vi "Project Directory Change Callback.vi"(4 "Variant":variant, 5 "Event Data":cluster{"sender":refnum<k24>, "e":refnum<k24>}, 6 "Control Ref":refnum<k24>, 7 "Event Common Data":T1) -> ()   [LabVIEW 2015, in "Editor.lvclass"]
uses:
  Editor.lvclass
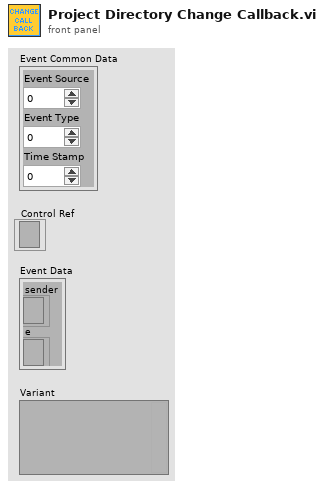
[diagram p1: front panel]
types:
  T1 = cluster{"Event Source":i32, "Event Type":u32, "Time Stamp":u32}
  T2 = cluster{"Event":enum16{"Changed", "Created", "Deleted", "Renamed", "Error"}, "Explorer Tree":refnum<vi>, "Path":path}
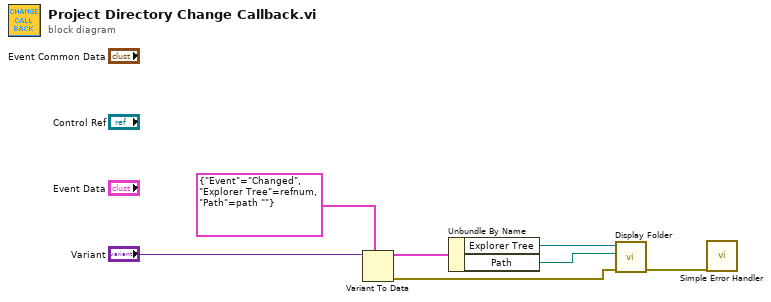
[diagram p0: block diagram]
diagram:
  n1 = Variant To Data(type=T2 {"Event"=enum."Changed", "Explorer Tree"=refnum, "Path"=path ""}, Variant="Variant") -> (data=w5:T2, error out=w2:errorcluster)  [unwired: 1 in]
  n2 = Unbundle By Name(w5) -> ("Explorer Tree"=w4:refnum<vi>, "Path"=w3:path)
  n3 = call "Display Folder.vi"("error in (no error)"=w2, "Folder in"=w3, "TreeControl in"=w4) -> ("error out"=w1:errorcluster)  [unwired: 6 in, 2 out]
  n4 = call <vilib>:"Simple Error Handler.vi"("error in (no error)"=w1) -> ()  [unwired: 4 in, 5 out]
